vi "Signale aléatoire décalé.vi"() -> ()   [LabVIEW 2014]
uses:
  <vilib>/Analysis/baseanly.llb/Mean (DBL).vi
  <vilib>/Analysis/NI_AALBase.lvlib
panel:
  out "Waveform Chart":cluster{"number: 0 to 1":dbl, "mean":dbl}(graph)
  in  "delai de boucle":dbl(knob) scale=0.0..2.0
  in  "stop":bool
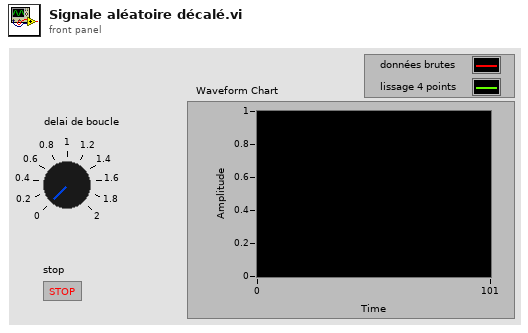
[diagram p1: front panel]
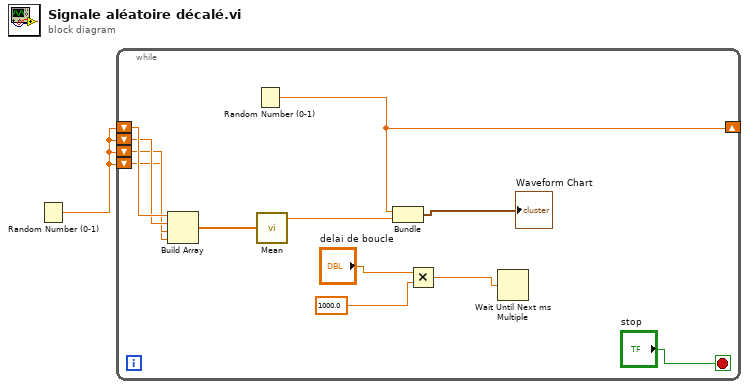
[diagram p0: block diagram]
diagram:
  n1 = Random Number (0-1)() -> (number: 0 to 1=w1:dbl)
  n2 = while {
    shift-right: [w2] -> _
    shift-left: w1 -> [w13]
    shift-left: w1 -> [w12]
    shift-left: w1 -> [w11]
    shift-left: w1 -> [w10]
    stop <- "stop" stop-if-true
    n3 = Build Array(w13, w12, w11, w10) -> (w8:dbl[])
    n4 = Random Number (0-1)() -> (number: 0 to 1=w2:dbl)
    n5 = call-poly <vilib>:"Mean.vi"("X"=w8) -> ("mean"=w7:dbl)  [unwired: 1 out]
    n6 = Bundle("number: 0 to 1"=w2, "mean"=w7) -> (→"Waveform Chart":cluster{"number: 0 to 1":dbl, "mean":dbl})  [unwired: 1 in]
    n7 = Multiply(x="delai de boucle", y=1000.0) -> (x*y=w3:dbl)
    n8 = Wait Until Next ms Multiple(millisecond multiple=w3) -> ()  [unwired: 1 out]
  }
